vi "Delete_Stored_Events.vi"(11 "user":i32) -> ()   [LabVIEW 2019]
panel:
  out "user":i32
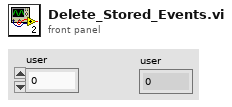
[diagram p1: front panel]
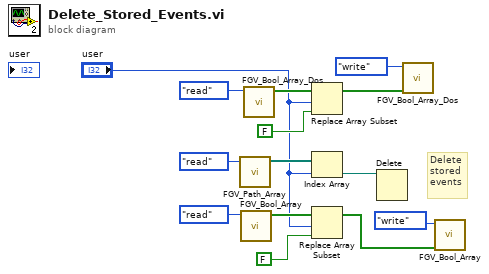
[diagram p0: block diagram]
diagram:
  # "Delete \nstored \nevents"
  n1 = call "FGV_Path_Array.vi"("Enum"=enum16{"read", "write"}."read" ("operation (0:open)")) -> ("path out"=w9:path[])  [unwired: 10 in]
  n2 = call "FGV_Bool_Array.vi"("Enum"=enum16{"read", "write"}."read") -> ("Array Out"=w6:bool[])  [unwired: 10 in]
  n3 = call "FGV_Bool_Array_Dos.vi"("Enum"=enum16{"read", "write"}."read" ("operation (0:open)")) -> ("Array Out"=w13:bool[])  [unwired: 10 in]
  n4 = Replace Array Subset(array=w13, new element=FALSE, index="user") -> (w11:bool[])
  n5 = Index Array(array=w9, index="user") -> (element=w8:path)
  n6 = Replace Array Subset(array=w6, new element=FALSE, index="user") -> (w4:bool[])
  n7 = Delete(path (use dialog)=w8) -> ()  [unwired: 4 in, 3 out]
  n8 = call "FGV_Bool_Array_Dos.vi"("Array In"=w11, "Enum"=enum16{"read", "write"}."write" ("operation (0:open)")) -> ()  [unwired: 9 in, 1 out]
  n9 = call "FGV_Bool_Array.vi"("Array In"=w4, "Enum"=enum16{"read", "write"}."write") -> ()  [unwired: 9 in, 1 out]
